vi "Practica_02.vi"() -> ()   [LabVIEW 2020]
uses:
  <vilib>/numeric/Random Number (Range) U64.vi
  <vilib>/numeric/sub_Random U32.vi
  <vilib>/express/express shared/transition.llb/Dynamic To Waveform Array.vi
  <vilib>/express/express signal manip/GetorSetDDTAttributes/Set DDT Attributes/SetT0.vi
  <vilib>/express/express shared/transition.llb/Waveform Array To Dynamic.vi
  <vilib>/express/express signal manip/GetorSetDDTAttributes/Set DDT Attributes/Set DDT Properties.xnode
panel:
  out "Dentro de rango":bool
  out "Número recibido":u64
  in  "Activar escritura de datos":bool=TRUE caption="Flush? (T)"
  out "Contador":u32=500
  in  "Stop":bool
  out "Grafica Filtro EMA":dbl(graph)
  out "Voltaje vs Tiempo":u64(graph)
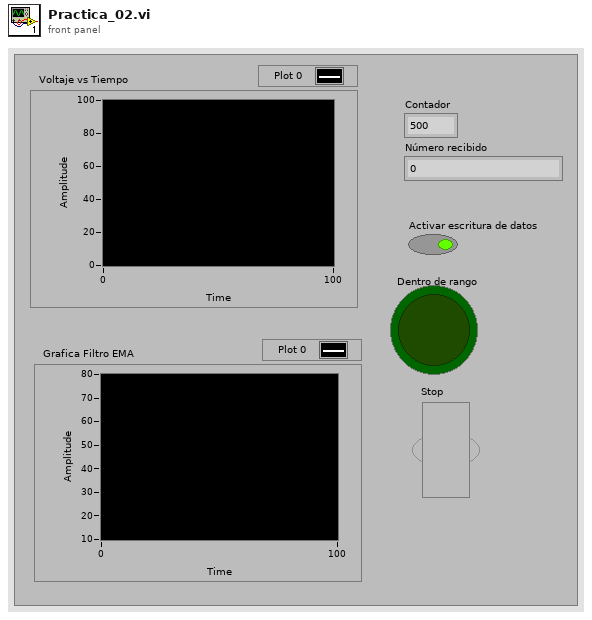
[diagram p1: front panel]
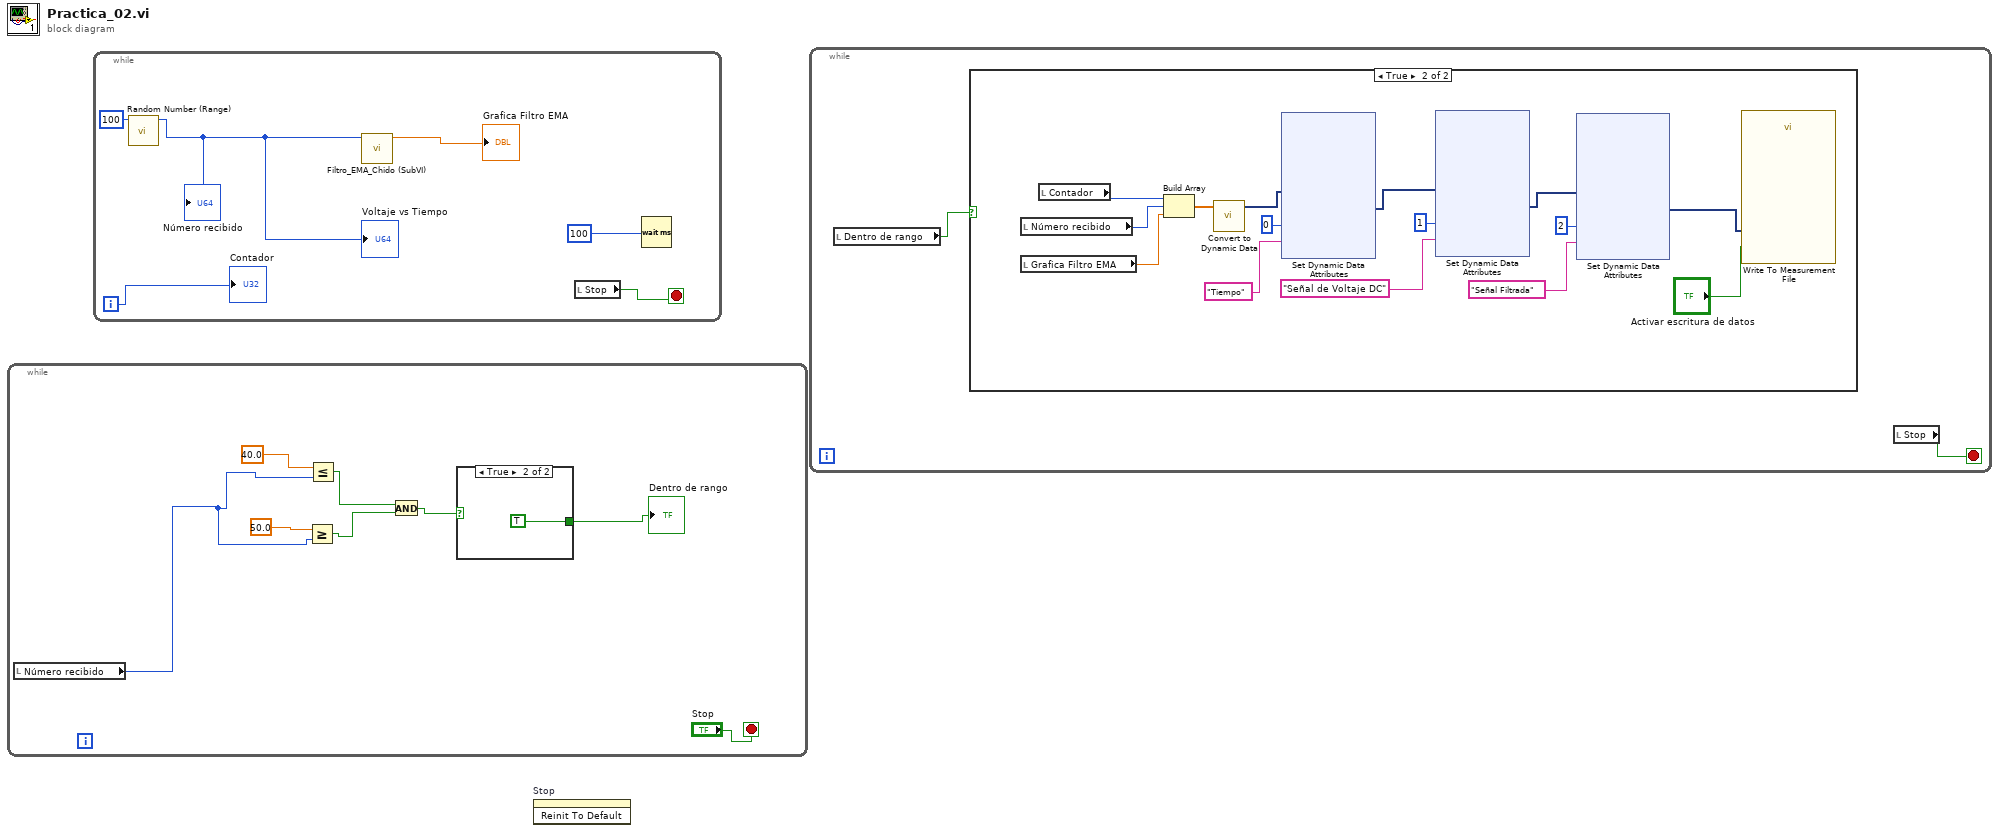
[diagram p0: block diagram]
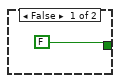
[diagram p3: hidden frame]
diagram:
  n1 = while {
    stop <- "Stop" stop-if-true
    n2 = local read "Número recibido"() -> (w1:u64)
    n3 = Greater Or Equal?(x=50.0, y=w1) -> (x >= y?=w3:bool)
    n4 = Less Or Equal?(x=40.0, y=w1) -> (x <= y?=w4:bool)
    n5 = And(x=w4, y=w3) -> (x .and. y?=w5:bool)
    n6 = case shown="True" w5 {
      tunnel: [FALSE TRUE] -> w2
      frame False {
      }
      frame True {
      }
    }
    "Dentro de rango" <- w2
  }
  n7 = while {
    i -> [w11]
    stop <- w14 stop-if-true
    n8 = call-poly <vilib>:"Random Number (Range).vi"("upper bound (100)"=u64 100) -> ("number"=w13:u64)  [unwired: 10 in]
    "Voltaje vs Tiempo" <- w13
    "Número recibido" <- w13
    n9 = call "Filtro_EMA_Chido (SubVI).vi"("Numeric in"=w13) -> ("Numeric out"=→"Grafica Filtro EMA":dbl)  [unwired: 10 in]
    n10 = local read "Stop"() -> (w14:bool)
    n11 = Wait (ms)(milliseconds to wait=u32 100) -> ()  [unwired: 1 out]
    "Contador" <- w11
  }
  n12 = invoke on="Stop" class="Bool (strict)" method="Reinit To Default"() -> ()  [unwired: 3 in, 3 out]
  n13 = while {
    stop <- w18 stop-if-true
    n14 = local read "Dentro de rango"() -> (w17:bool)
    n15 = case shown="True" w17 {
      frame False {
      }
      frame True {
        n16 = local read "Número recibido"() -> (w26:u64)
        n17 = local read "Grafica Filtro EMA"() -> (w25:dbl)
        n18 = local read "Contador"() -> (w22:u32)
        n19 = Build Array(w22, w26, w25) -> (w27:dbl[])
        n20 = call "Convert to Dynamic Data"("Array"=w27) -> ("Dynamic Data Type"=w24:dynamicdata)  [unwired: 3 in]
        n21 = xnode "Set Dynamic Data Attributes"("Signals In"=w24, "Signal Index"=0, "Signal Name"="Tiempo") -> ("Signals Out"=w32:dynamicdata)  [unwired: 1 in, 1 out]
        n22 = xnode "Set Dynamic Data Attributes"("Signals In"=w32, "Signal Index"=1, "Signal Name"="Señal de Voltaje DC") -> ("Signals Out"=w30:dynamicdata)  [unwired: 1 in, 1 out]
        n23 = xnode "Set Dynamic Data Attributes"("Signals In"=w30, "Signal Index"=2, "Signal Name"="Señal Filtrada") -> ("Signals Out"=w28:dynamicdata)  [unwired: 1 in, 1 out]
        n24 = call "Write To Measurement File"("Signals"=w28, "Flush? (T)"="Activar escritura de datos") -> ()  [unwired: 15 in, 3 out]
      }
    }
    n25 = local read "Stop"() -> (w18:bool)
  }
